vi "Close.vi"(8 "error in (no error)":errorcluster, 11 "Communication in":refnum<class "IP_Communication.lvclass">) -> (0 "error out":errorcluster, 3 "Communication out":refnum<class "IP_Communication.lvclass">)   [LabVIEW 2020, in "Communication Classes.lvlib" / "IP_Communication.lvclass"]
uses:
  IP_Communication.lvclass
  IP_Communication.lvclass/IP_Communication.ctl
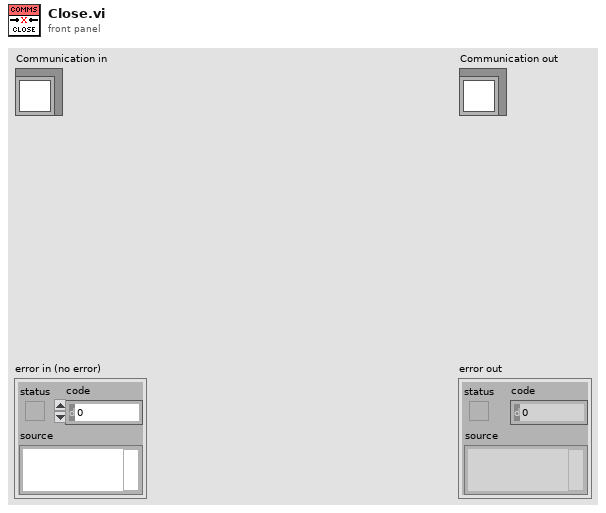
[diagram p1: front panel]
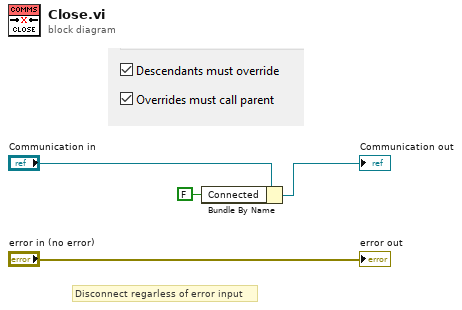
[diagram p0: block diagram]
diagram:
  # "Disconnect regarless of error input"
  n1 = Bundle By Name(cluster="Communication in", "Connected"=FALSE) -> (→"Communication out":refnum<class "IP_Communication.lvclass">)
  "error out" <- "error in (no error)"
